vi "nominal_channel_writer.write_batches_string.vi"(7 "Tags":cluster{"Name":string, "Value":string}[](array[cluster]), 8 "error in":errorcluster, 9 "batches":T1(array[cluster]), 10 "Data Source RID":string, 11 "Nominal Client in":refnum<class "Nominal Client.lvclass">) -> (0 "error out":errorcluster, 2 "Response body":string, 3 "Nominal Client out":refnum<class "Nominal Client.lvclass">)   [LabVIEW 2018, in "Nominal Client.lvclass"]
doc: "Synchronously writes batches of records to a Nominal data source.\n\nTAGS:\nThis is a malleable VI (VIM) that will accept:\n- Map: Name (String) -> Value (String)\n- Array of Clusters: {Name (String), Value (String)}\n- Cluster: {Array of Names (String), Array of Values (String)}"
uses:
  Nominal Client.lvclass
  Nominal Client.lvclass/Nominal Client.ctl
  cdde0a50-1f2d-45b6-8c5c-67b334d1f5bb.vi
  2aaf4cd1-b7d0-4e89-be55-e948b2020e34.vi
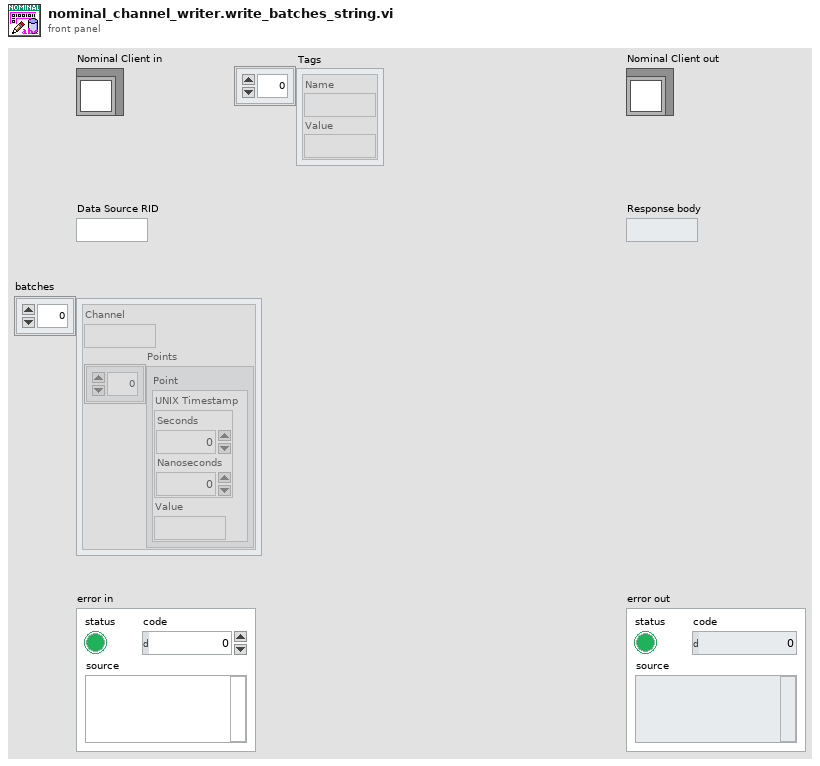
[diagram p1: front panel]
types:
  T1 = cluster{"Channel":string, "Points":cluster{"UNIX Timestamp":cluster{"Seconds":i64, "Nanoseconds":i64}, "Value":string}[]}[]
  T2 = cluster{"batches":cluster{"channel":string, "points":cluster{"type":string, "string":cluster{"timestamp":cluster{"seconds":i32, "nanos":i32}, "value":string}[]}}[], "tags":variant, "dataSourceRid":string}
  T3 = cluster{"UNIX Timestamp":cluster{"Seconds":i64, "Nanoseconds":i64}, "Value":string}[]
  T4 = cluster{"type":string, "Points":cluster{"UNIX Timestamp":cluster{"Seconds":i64, "Nanoseconds":i64}, "Value":string}[]}
  T5 = cluster{"Channel":string, cluster{"type":string, "Points":cluster{"UNIX Timestamp":cluster{"Seconds":i64, "Nanoseconds":i64}, "Value":string}[]}}
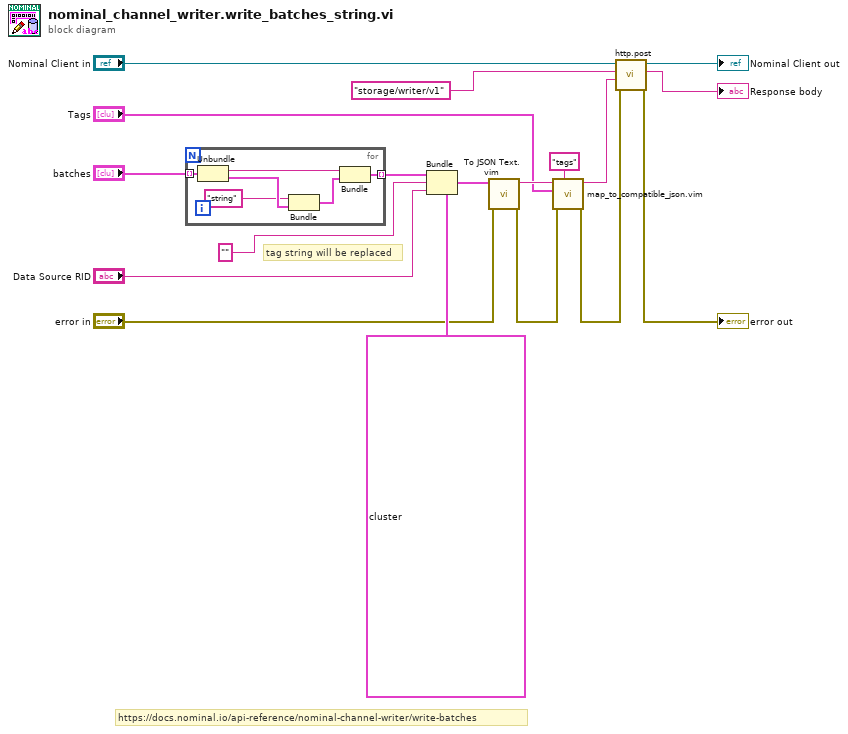
[diagram p0: block diagram]
diagram:
  # "tag string will be replaced"
  # "https://docs.nominal.io/api-reference/nominal-channel-writer/write-batches"
  n1 = for {
    tunnel: "batches" -> [w24] mode=indexing
    tunnel: [w19] -> w3 mode=indexing
    n2 = Unbundle(w24) -> ("Channel"=w23:string, "Points"=w22:T3)
    n3 = Bundle("type"="string", "Points"=w22) -> (w20:T4)  [unwired: 1 in]
    n4 = Bundle("Channel"=w23, w20) -> (w19:T5)  [unwired: 1 in]
  }
  n5 = Bundle(cluster=T2 {"batches"=[], "tags"=variant, "dataSourceRid"=""} ("output cluster"), "batches"=w3, "tags"="", "dataSourceRid"="Data Source RID") -> (w11:T2)
  n6 = call "To JSON Text.vim"("error in (no error)"="error in", "Anything"=w11) -> ("error out"=w7:errorcluster, "<JSON>"=w9:string)  [unwired: 8 in]
  n7 = call "map_to_compatible_json.vim"("JSON Path"="tags", "error in"=w7, "Tags"="Tags", "JSON in"=w9) -> ("error out"=w6:errorcluster, "JSON out"=w8:string)  [unwired: 6 in]
  n8 = call "http.post.vi"("error in"=w6, "Request body"=w8, "Path"="storage/writer/v1", "Nominal Client in"="Nominal Client in") -> ("error out"=→"error out":errorcluster, "Response"=→"Response body":string, "Nominal Client out"=→"Nominal Client out":refnum<class "Nominal Client.lvclass">)  [unwired: 4 in, 1 out]
